vi "HTTPBasicAccessAuthentication.vi"(9 "Realm":string, 10 "Base64 user:pass":string, 11 "LabVIEW Web Service Request":refnum<class "Web Request.lvclass">) -> (3 "LabVIEW Web Service Request out":refnum<class "Web Request.lvclass">)   [LabVIEW 2013]
doc: "Basic access authentication for any RESTful web service method.\nUsername and password have to be combined to a string \"username:password\" and Base64-encoded."
uses:
  <vilib>/wsapi/Web Request.lvclass
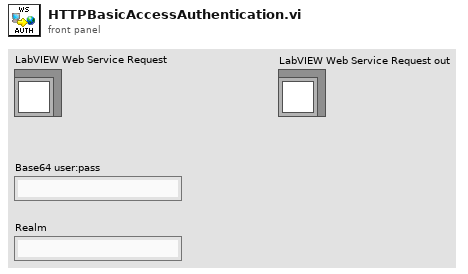
[diagram p1: front panel]
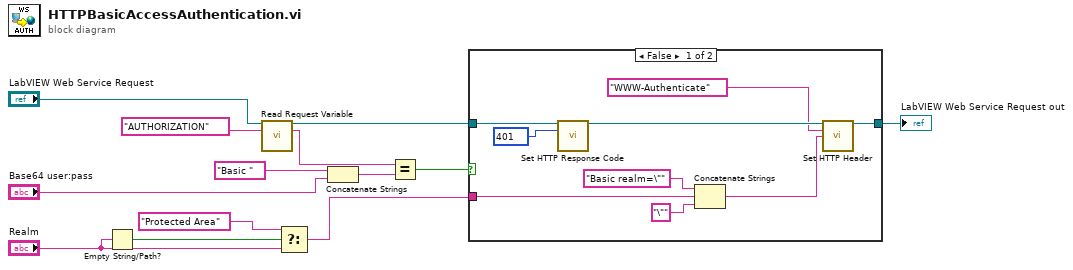
[diagram p0: block diagram]
diagram:
  n1 = Empty String/Path?(string/path="Realm") -> (empty?=w4:bool)
  n2 = call <vilib>:"Read Request Variable.vi"("LabVIEW Web Service Request"="LabVIEW Web Service Request", "variable name"="AUTHORIZATION" ("header")) -> ("LabVIEW Web Service Request out"=w6:refnum<class "Web Request.lvclass">, "value"=w11:string)  [unwired: 11 in, 1 out]
  n3 = Select(t="Protected Area", s=w4, f="Realm") -> (s? t:f=w1:string)
  n4 = Concatenate Strings("Basic ", "Base64 user:pass") -> (w8:string)
  n5 = Equal?(x=w11, y=w8) -> (x = y?=w7:bool)
  n6 = case shown="False" w7 {
    tunnel: w6 -> [w22 w23]
    tunnel: [w18 w23] -> w5
    tunnel: w1 -> [w16 _]
    frame False {
      w19 = 401 items=["100"=100, "101"=101, "200"=200, "201"=201, "202"=202, "203"=203, "204"=204, "205"=205, "206"=206, "300"=300, "301"=301, "302"=302, "303"=303, "304"=304, "305"=305, "306"=306, "307"=307, "400"=400, "401"=401, "402"=402, "403"=403, "404"=404, "405"=405, "406"=406, "407"=407, "408"=408, "409"=409, "410"=410, "411"=411, "412"=412, "413"=413, "414"=414, "415"=415, "416"=416, "417"=417, "500"=500, "501"=501, "502"=502, "503"=503, "504"=504, "505"=505] ("response code (200)")
      n7 = call <vilib>:"Set HTTP Response Code.vi"("LabVIEW Web Service Request"=w22, "response code (200)"=w19) -> ("LabVIEW Web Service Request out"=w21:refnum<class "Web Request.lvclass">)  [unwired: 12 in, 1 out]
      n8 = Concatenate Strings("Basic realm=\"" ("header"), w16, "\"" ("string")) -> (w14:string)
      n9 = call <vilib>:"Set HTTP Header.vi"("LabVIEW Web Service Request"=w21, "header"="WWW-Authenticate", "header value"=w14) -> ("LabVIEW Web Service Request out"=w18:refnum<class "Web Request.lvclass">)  [unwired: 11 in, 1 out]
    }
    frame True {
    }
  }
  "LabVIEW Web Service Request out" <- w5
